vi "Motic Get Type.vi"(8 "error in (no error)":errorcluster, 11 "camera":i32) -> (0 "error out":errorcluster, 2 "camera type":u32(ring), 3 "camera out":i32)   [LabVIEW 2012, in "MoticApi.lvlib"]
doc: "MOTICAPI MUCam_Type Motic_GetType(MUCam_Handle camera);"
uses:
  MoticApi.lvlib
  MoticApi.dll
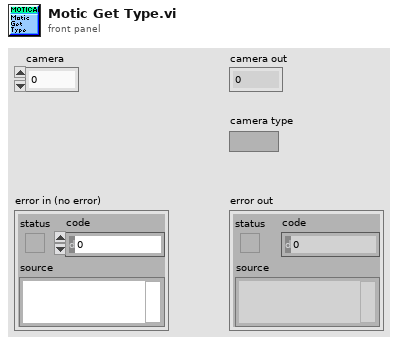
[diagram p1: front panel]
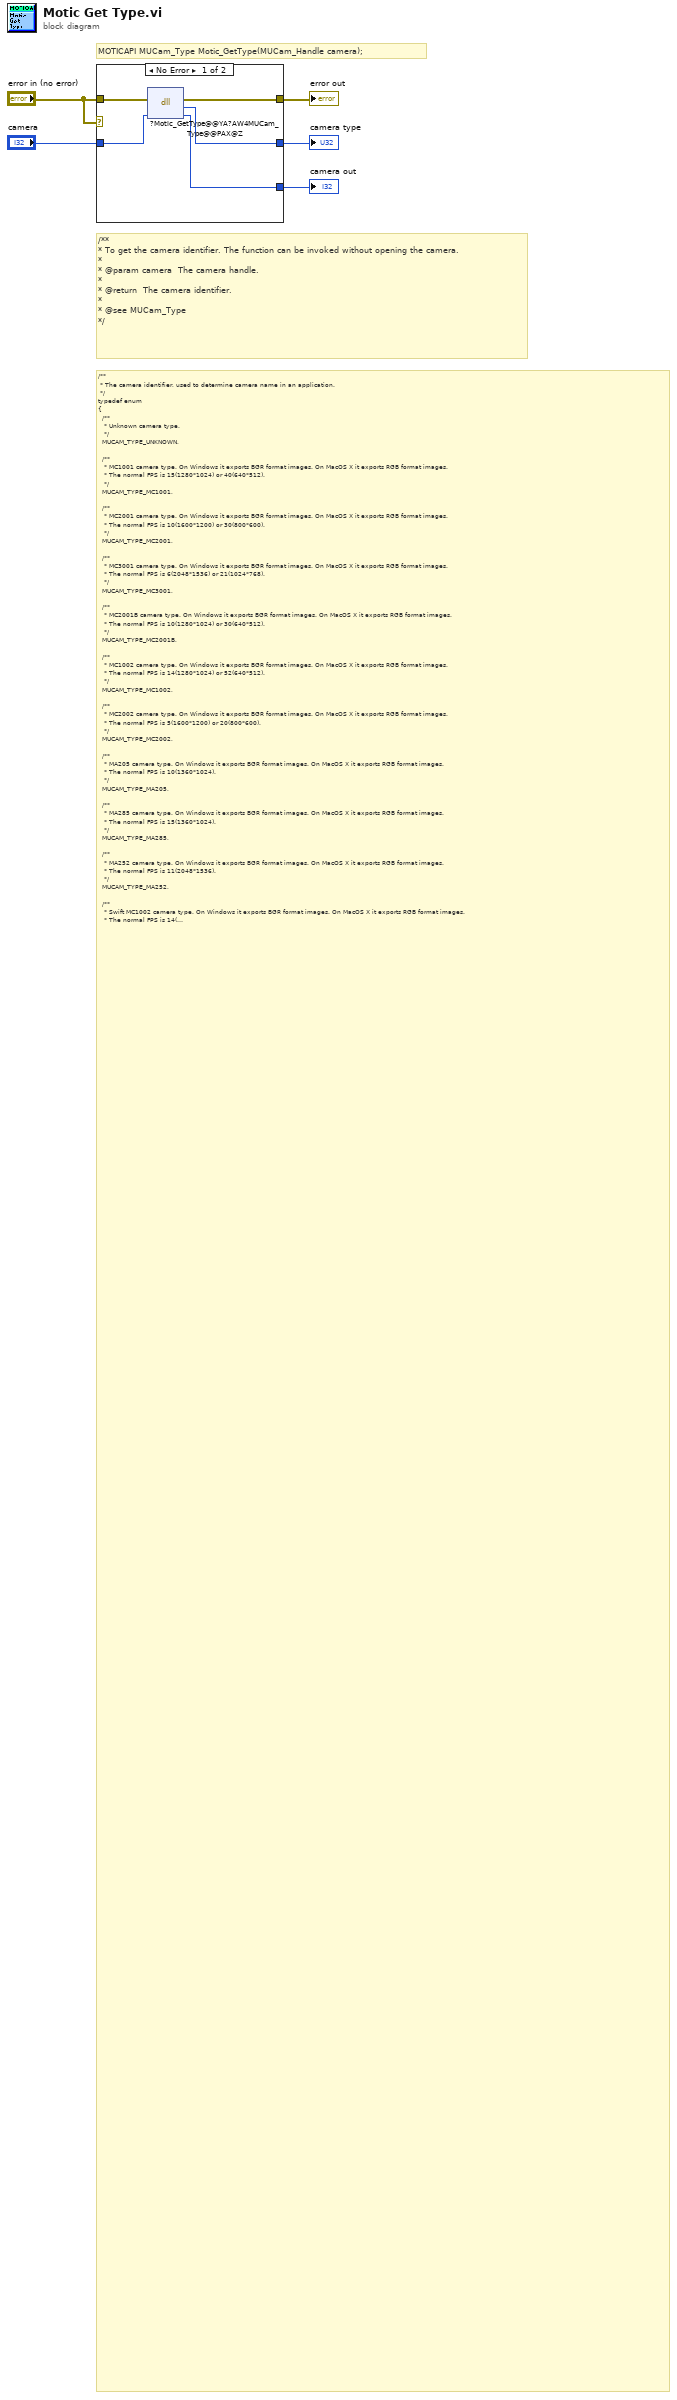
[diagram p0: block diagram]
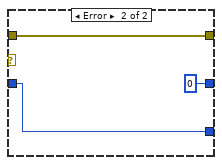
[diagram p2: hidden frame]
diagram:
  # "/**\n * The camera identifier, used to determine camera name in an application.\n */\ntypedef enum\n{\n  /**\n   * Unknown camera type.\n   */\n  MUCAM_TYPE_UNKNOWN,\n\n  /**\n   * MC1001 camera type. On Windows it exports BGR format images. On MacOS X it exports RGB format images.\n   * The normal FPS is 15(1280*1024) or 40(640*512).\n   */\n  MUCAM_TYPE_MC1001,\n\n  /**\n   * MC2001 camera type. On Windows it exports BGR format images. On MacOS X it exports RGB format images.\n   * The normal FPS is 10(1600*1200) or 30(800*600).\n   */\n  MUCAM_TYPE_MC2001,\n\n  /**\n   * MC3001 camera type. On Windows it exports BGR format images. On MacOS X it exports RGB format images.\n   * The normal FPS is 6(2048*1536) or 21(1024*768).\n   */\n  MUCAM_TYPE_MC3001,\n\n  /**\n   * MC2001B camera type. On Windows it exports BGR format images. On MacOS X it exports RGB format images.\n   * The normal FPS is 10(1280*1024) or 30(640*512).\n   */\n  MUCAM_TYPE_MC2001B,\n\n  /**\n   * MC1002 camera type. On Windows it exports BGR format images. On MacOS X it exports RGB format images.\n   * The normal FPS is 14(1280*1024) or 52(640*512).\n   */\n  MUCAM_TYPE_MC1002,\n\n  /**\n   * MC2002 camera type. On Windows it exports BGR format images. On MacOS X it exports RGB format images.\n   * The normal FPS is 5(1600*1200) or 20(800*600).\n   */\n  MUCAM_TYPE_MC2002,\n\n  /**\n   * MA205 camera type. On Windows it exports BGR format images. On MacOS X it exports RGB format images.\n   * The normal FPS is 10(1360*1024).\n   */\n  MUCAM_TYPE_MA205,\n\n  /**\n   * MA285 camera type. On Windows it exports BGR format images. On MacOS X it exports RGB format images.\n   * The normal FPS is 15(1360*1024).\n   */\n  MUCAM_TYPE_MA285,\n\n  /**\n   * MA252 camera type. On Windows it exports BGR format images. On MacOS X it exports RGB format images.\n   * The normal FPS is 11(2048*1536).\n   */\n  MUCAM_TYPE_MA252,\n\n  /**\n   * Swift MC1002 camera type. On Windows it exports BGR format images. On MacOS X it exports RGB format images.\n   * The normal FPS is 14(1280*1024) or 52(640*512).\n   */\n  MUCAM_TYPE_SWIFT_MC1002,\n\n  /**\n   *\n   * Undocumented.\n   *\n   * @deprecated Since MA252 added.\n   */\n  MUCAM_TYPE_MD3300,\n\n  /**\n   * MC5001 camera type. On Windows it exports BGR format images. On MacOS X it exports RGB format images.\n   * The normal FPS is 7(2592*1944) or 20(1296*972).\n   */\n  MUCAM_TYPE_MC5001,\n\n  /**\n   * MC3111 camera type. On Windows it exports BGR format images. On MacOS X it exports RGB format images\n   * the normal FPS is 13(1280*1024) or 40(640*480)\n   */\n  MUCAM_TYPE_MC3111,\n\n  /**\n   * MC3222 camera type. On Windows it exports BGR format images. On MacOS X it exports RGB format images\n   * the normal FPS is 10(1600*1200) or 30(800*600)\n   */\n  MUCAM_TYPE_MC3222,\n\n  /**\n   * MC3022 camera type. On Windows it exports BGR format images. On MacOS X it exports RGB format images\n   * the normal FPS is 7(1600*1200) or 20(800*600) \n   */\n  MUCAM_TYPE_MC3022,\n\n  /** \n   * Swift MC3001 camera type. On Windows it exports BGR format images. On MacOS X it exports RGB format images.\n   * The normal FPS is 6(2048*1536) or 21(1024*768).\n   */\n  MUCAM_TYPE_SWIFT_MC3001,\n\n  /**\n  * Swift MC3222 camera type. On Windows it exports BGR format images. On MacOS X it exports RGB format images\n  * the normal FPS is 10(1600*1200) or 30(800*600)\n  */\n  MUCAM_TYPE_SWIFT_MC3222,\n\n  /**\n  * Swift MC3111 camera type. On Windows it exports BGR format images. On MacOS X it exports RGB format images\n  * the normal FPS is 13(1280*1024) or 40(640*480)\n  */\n  MUCAM_TYPE_SWIFT_MC3111,\n \n  /**\n  * MA282 camera type. On Windows it exports BGR format images. On MacOS X it exports RGB format images.\n  * The normal FPS is 6(2560*1920).\n  */\n  MUCAM_TYPE_MA282,\n\n  /**\n   * @brief MC352+ Camrea\n   *  \n   * Undocumented. Not available at present.\n   */\n  MUCAM_TYPE_MC352PLUS,\n\n  /**\n   * @brief MC3521\n   *\n   * Undocumented. Not available at present.   \n   */\n  MUCAM_TYPE_MC3521,\n\n  /**   \n   * MC10M camera type. On Windows/Linux it exports BGR format images. On MacOS X it exports RGB format images.\n   * The normal FPS is 2.2(3664*2748) or 8.5(1832*1374) or 30(916*686).\n   */\n  MUCAM_TYPE_MC10M\n\n} MUCam_Type;"
  # "/**\n* To get the camera identifier. The function can be invoked without opening the camera.\n*\n* @param camera  The camera handle.\n*\n* @return  The camera identifier.\n*\n* @see MUCam_Type\n*/"
  # "MOTICAPI MUCam_Type Motic_GetType(MUCam_Handle camera);"
  n1 = case shown="No Error" "error in (no error)" {
    tunnel: [w10 u32 0 ("return type")] -> w5
    tunnel: "camera" -> [w9 w12]
    tunnel: [w8 w12] -> w3
    tunnel: "error in (no error)" -> [w7 w13]
    tunnel: [w6 w13] -> w2
    frame No Error {
      n2 = dll-call lib="C:/Users/TTS-Digital/Desktop/MoticApi/MoticApi_git/MoticApi/MoticApi.*" fn="?Motic_GetType@@YA?AW4MUCam_Type@@PAX@Z"(error in=w7, "camera"=w9) -> (error out=w6:errorcluster, "return type"=w10:u32, "camera"=w8:i32)  [unwired: 2 in, 1 out]
    }
    frame Error {
    }
  }
  "camera type" <- w5
  "camera out" <- w3
  "error out" <- w2
